vi "XPS Controller.vi"(4 "Axis 2":string="Group7", 5 "Axis 1":string="Group2", 7 "Controller Address":string="192.168.254.254", 9 "Axis 2 \ninverted?":bool=TRUE, 10 "Axis 1 \ninverted?":bool=TRUE) -> ()   [LabVIEW 2016]
uses:
  <vilib>/Utility/miscctls.llb/LVMinMaxIncTypeDef.ctl
panel:
  in  "Data Entry Limits":T1
  in  "Axis Initial Parameters":T2={"Velocity (units/seconds)"=1.0, "Acceleration (units/seconds²)"=20.0, "Minimum Jerk Time (seconds)"=0.005, "Maximum Jerk Time (seconds)"=0.009} {"Maximum Jerk Time (seconds)" format="%.6e"; "Minimum Jerk Time (seconds)" format="%.6e"; "Acceleration (units/seconds²)" format="%.6e"; "Velocity (units/seconds)" format="%.6e"}
  in  "Mode selector":bool
  in  "Axis 2 Velocity (slow)\nmm/s":dbl=1.0 min=0.0 max=10.0 step=0.0001
  in  "Axis 2 Velocity (fast)\nmm/s":dbl=5.0 min=0.0 max=10.0 step=0.0001
  in  "Velocity (slow)":dbl=1.0 min=0.0 max=5.0 step=0.0001
  in  "Velocity (fast)":dbl=5.0 min=0.0 max=5.0 step=0.0001
  in  "Refresh Time":u32=100 min=50 max=10000 step=1
  in  "Tab Control":enum32{"JOG MODE", "MOVE MODE"}(tab)
  in  "Axis 1 negative":bool
  in  "Axis 1 negative fast":bool
  in  "Axis 1 Positive":bool
  in  "Axis 1 Positive fast":bool
  in  "Axis 2 negative":bool
  in  "Axis 2 negative fast":bool
  in  "Axis 2 Positive":bool
  in  "Axis 2 Positive fast":bool
  in  "Absolute":dbl=5.0 min=0.0 max=50.0
  in  "Absolute Axis 2":dbl=5.0 min=-75.0 max=75.0
  in  "Axis 1 move absolute":bool
  in  "Axis 2 move absolute":bool
  in  "Relative":dbl=1.0 min=-50.0 max=50.0
  in  "Relative Axis 2":dbl=1.0 min=-150.0 max=150.0
  in  "Axis 1 move relative":bool
  in  "Axis 2 move relative":bool
  out "Axis 1 Model":string
  out "Axis 2 Model":string
  in  "stop 2":bool
  out "Axis 2 position":dbl format="%.10f"
  out "Axis 2 Status":string
  out "Axis 1 position":dbl format="%.10f"
  out "Axis 1 Status":string
  in  "Motion parameter":T3={"Velocity (units/s)"=5.0, "Acceleration (units/s²)"=20.0} {"Acceleration (units/s²)" format="%.6f"; "Velocity (units/s)" format="%.6f"}
  in  "stop":bool
  # "Axis 1"
  # "Axis 2"
  # "msec"
  # "Axis 1"
  # "Axis 2"
  # "Axis 1"
  # "Axis 2"
  # "Absolute"
  # "Relative"
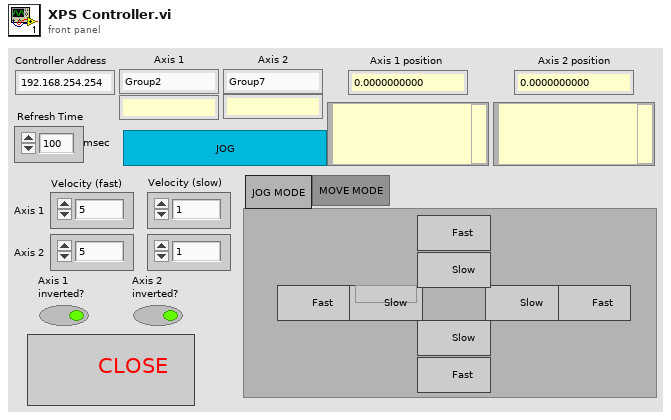
[diagram p1: front panel]
types:
  T1 = typedef "LVMinMaxIncTypeDef.ctl" = cluster{"Minimum":dbl, "Maximum":dbl, "Increment":dbl}
  T2 = cluster{"Velocity (units/seconds)":dbl, "Acceleration (units/seconds²)":dbl, "Minimum Jerk Time (seconds)":dbl, "Maximum Jerk Time (seconds)":dbl}
  T3 = cluster{"Velocity (units/s)":dbl, "Acceleration (units/s²)":dbl}
  T4 = enum32{"Page Enabled", "Page Disabled", "Page Disabled & Grayed"}
  T5 = cluster{"connection TCP":refnum<k5>, "LogTo File":bool, "Log File refnum":refnum<file>, "no error if error log":bool}
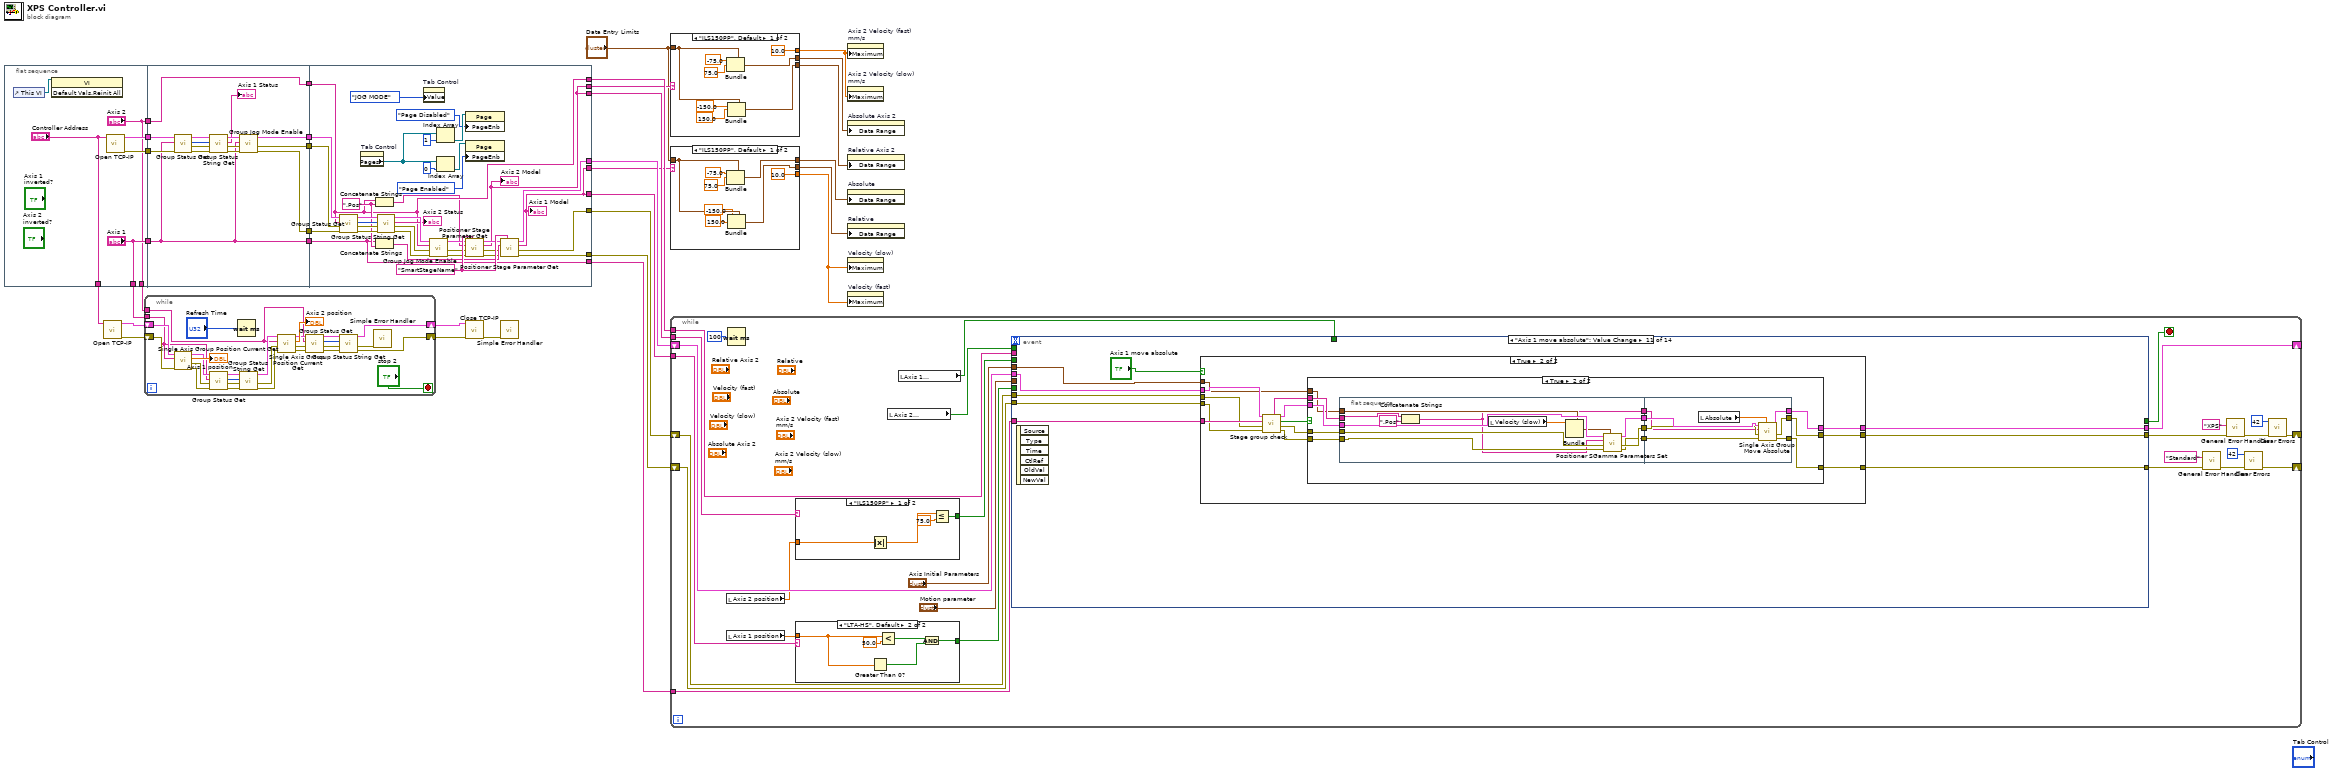
[diagram p0: block diagram]
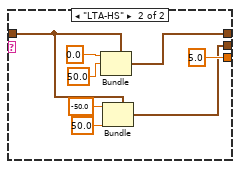
[diagram p2: hidden frame]
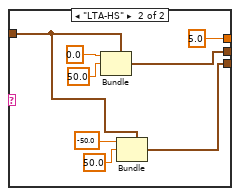
[diagram p3: hidden frame]
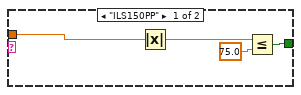
[diagram p4: hidden frame]
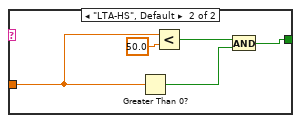
[diagram p5: hidden frame]
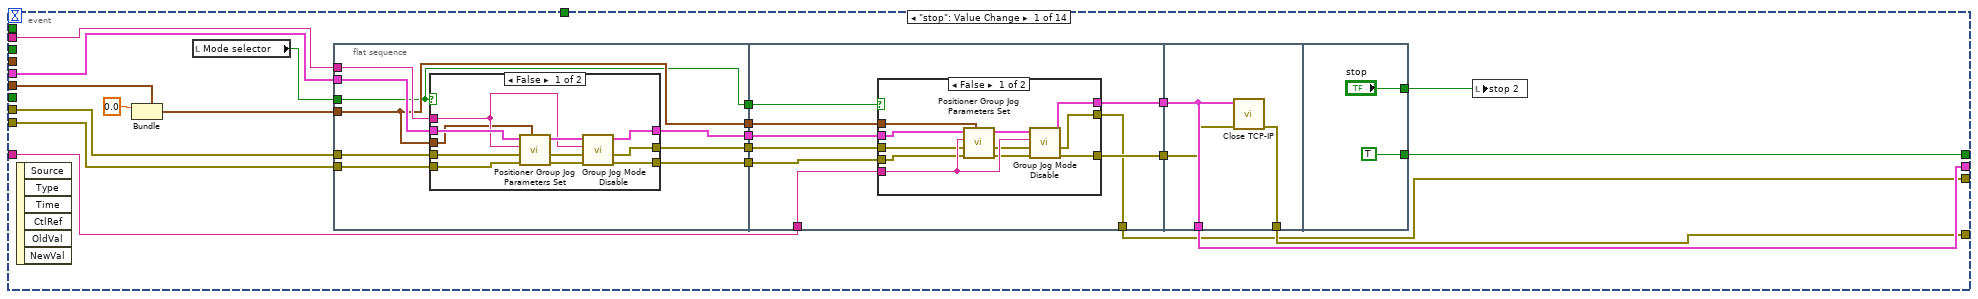
[diagram p6: hidden frame]
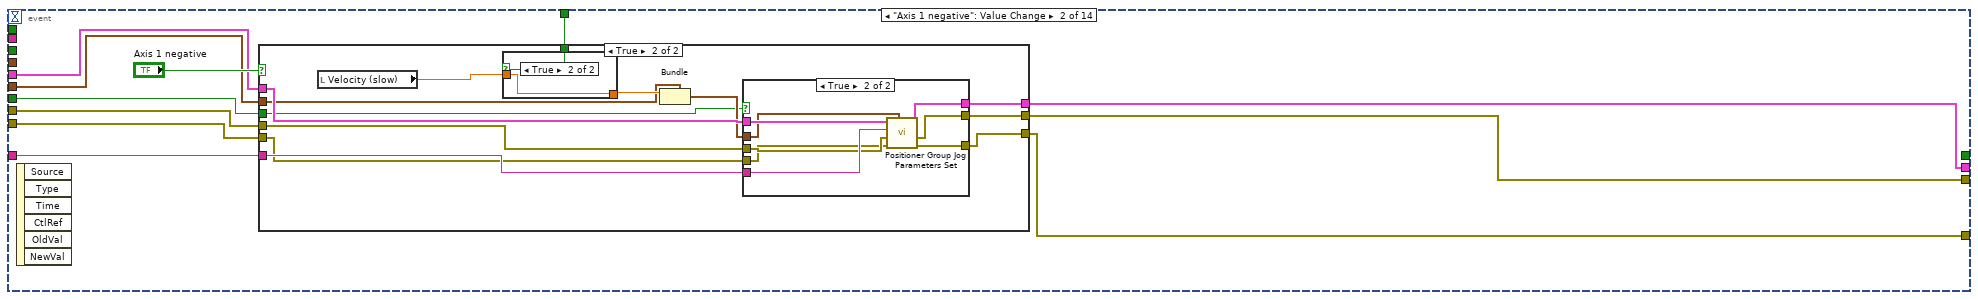
[diagram p9: hidden frame]
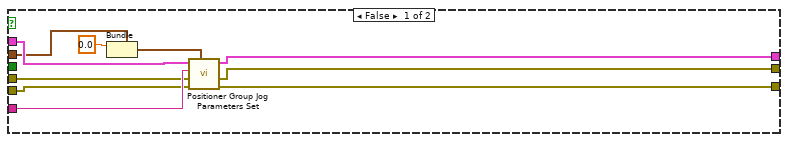
[diagram p10: hidden frame]
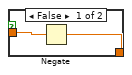
[diagram p11: hidden frame]
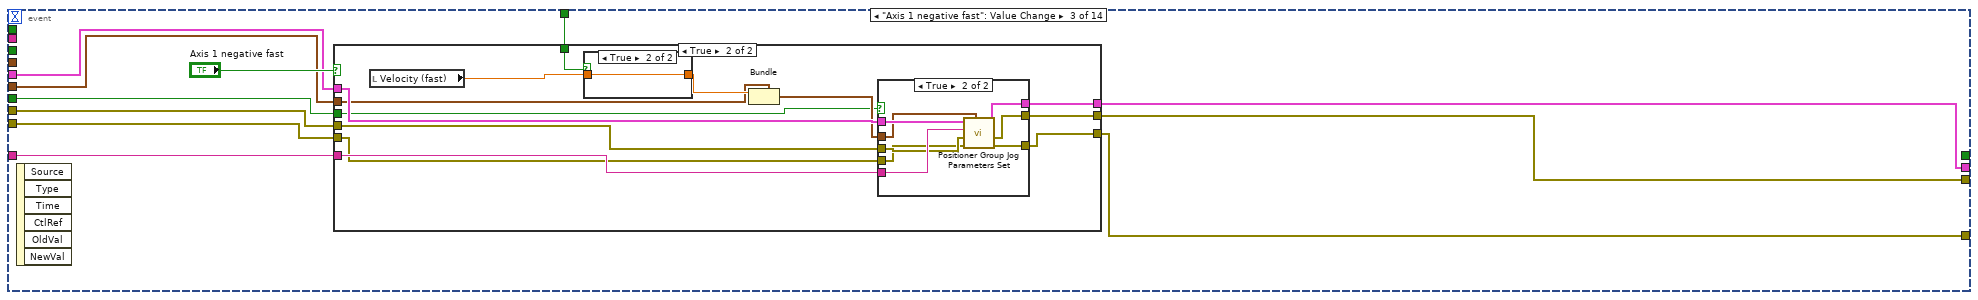
[diagram p13: hidden frame]
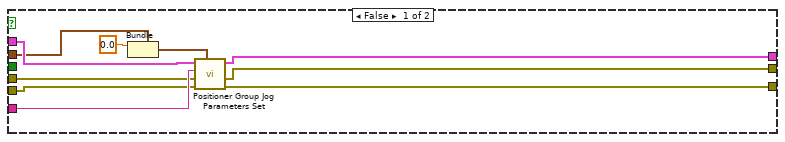
[diagram p14: hidden frame]
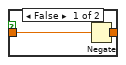
[diagram p15: hidden frame]
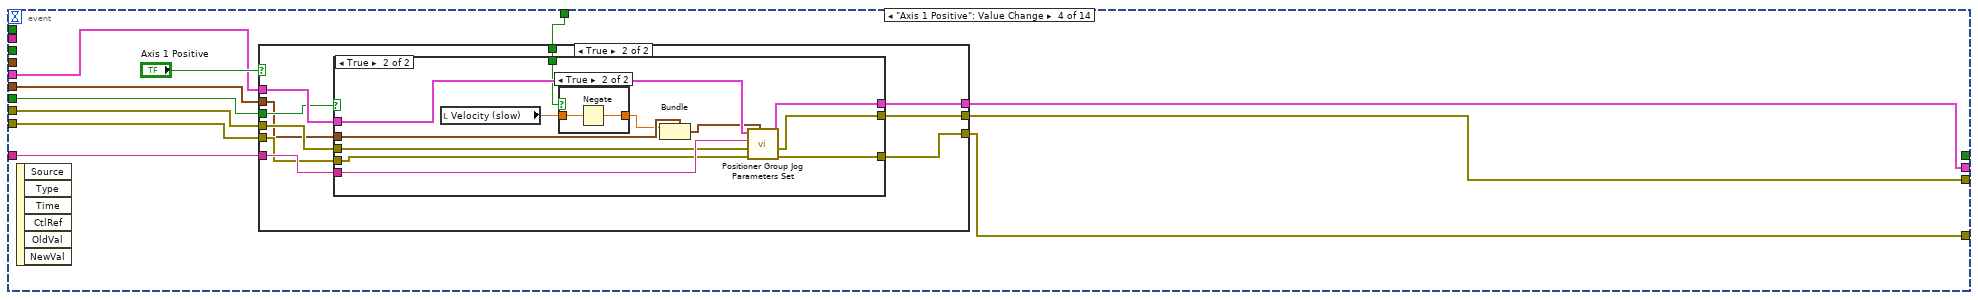
[diagram p17: hidden frame]
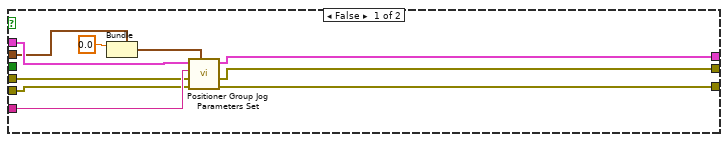
[diagram p18: hidden frame]
diagram:
  n1 = flat-sequence {
    tunnel: ["Axis 1"] -> w30
    tunnel: [w38] -> w29
    tunnel: [w37] -> w28
    tunnel: ["Axis 2"] -> w27
    tunnel: ["Controller Address"] -> w21
    tunnel: ["Axis 1"] -> w16
    tunnel: ["Axis 2"] -> w15
    tunnel: [w54] -> w33
    tunnel: [w53] -> w32
    tunnel: [w52] -> w31
    tunnel: w30 -> [w41]
    tunnel: w29 -> [w47]
    tunnel: w28 -> [w46]
    tunnel: w27 -> [w40]
    tunnel: [w40] -> w26
    tunnel: [w41] -> w24
    tunnel: w33 -> [w87]
    tunnel: w32 -> [w81]
    tunnel: w31 -> [w82]
    tunnel: w26 -> [w73]
    tunnel: w24 -> [w74]
    tunnel: [w65] -> w13
    tunnel: [w76] -> w25
    tunnel: [w74] -> w22
    tunnel: [w73] -> w23
    tunnel: [w68] -> w12
    tunnel: [w63] -> w11
    tunnel: [w64] -> w10
    tunnel: [w64] -> w9
    tunnel: [w63] -> w8
    frame #0 {
      n2 = control-ref of="This VI"() -> (w39:refnum<vi>)
      n3 = invoke class="VI" method="Default Vals.Reinit All"(reference=w39) -> ()  [unwired: 2 in, 3 out]
      n4 = call <userlib>:"Open TCP-IP.vi"("IP address"="Controller Address") -> ("error out"=w38:errorcluster, "Connection ID"=w37:T5)  [unwired: 5 in, 4 out]
    }
    frame #1 {
      n5 = call <userlib>:"Group Status Get.vi"("error in (no error)"=w47, "Group Name (250 c max)"=w41, "connection ID in"=w46) -> ("error out"=w50:errorcluster, "XPS error out"=w51:errorcluster, "Status"=w49:i32, "connection ID out"=w45:T5)  [unwired: 5 in]
      n6 = call <userlib>:"Group Status String Get.vi"("error in (no error)"=w50, "XPS error in (no error)"=w51, "Status #"=w49, "connection ID in"=w45) -> ("error out"=w44:errorcluster, "XPS error out"=w43:errorcluster, "Group Status String"=→"Axis 1 Status":string, "connection ID out"=w48:T5)  [unwired: 4 in]
      n7 = call <userlib>:"Group Jog Mode Enable.vi"("error in (no error)"=w44, "XPS error in (no error)"=w43, "Group Name (250 c max)"=w41, "connection ID in"=w48) -> ("error out"=w52:errorcluster, "XPS error out"=w53:errorcluster, "connection ID out"=w54:T5)  [unwired: 5 in]
    }
    frame #2 {
      w75 = ".Pos" ("string")
      w79 = "SmartStageName" ("Parameter Name (250 c max)")
      n8 = call <userlib>:"Group Status Get.vi"("error in (no error)"=w82, "XPS error in (no error)"=w81, "Group Name (250 c max)"=w73, "connection ID in"=w87) -> ("error out"=w89:errorcluster, "XPS error out"=w90:errorcluster, "Status"=w88:i32, "connection ID out"=w86:T5)  [unwired: 4 in]
      n9 = property on="Tab Control" class="TabCtl (strict)"() -> ("Pages"=w56:refnum<vi>[])  [unwired: 2 in, 2 out]
      n10 = Concatenate Strings(w73, w75) -> (w72:string)
      n11 = Concatenate Strings(w74, w75) -> (w71:string)
      n12 = call <userlib>:"Group Status String Get.vi"("error in (no error)"=w89, "XPS error in (no error)"=w90, "Status #"=w88, "connection ID in"=w86) -> ("error out"=w84:errorcluster, "XPS error out"=w83:errorcluster, "Group Status String"=→"Axis 2 Status":string, "connection ID out"=w85:T5)  [unwired: 4 in]
      n13 = property on="Tab Control" class="TabCtl (strict)"("Value"=enum32{"JOG MODE", "MOVE MODE"}."JOG MODE" ("Tab Control")) -> ()  [unwired: 2 in, 2 out]
      n14 = call <userlib>:"Group Jog Mode Enable.vi"("error in (no error)"=w84, "XPS error in (no error)"=w83, "Group Name (250 c max)"=w73, "connection ID in"=w85) -> ("error out"=w70:errorcluster, "XPS error out"=w67:errorcluster, "connection ID out"=w78:T5)  [unwired: 5 in]
      n15 = Index Array(array=w56, index=1) -> (element=w58:refnum<vi>)
      n16 = Index Array(array=w56, index=0) -> (element=w60:refnum<vi>)
      n17 = property class="Page"(reference=w58, "PageEnb"=T4."Page Disabled" ("Page Enabled State")) -> ()  [unwired: 1 in, 2 out]
      n18 = property class="Page"(reference=w60, "PageEnb"=T4."Page Enabled" ("Page Enabled State")) -> ()  [unwired: 1 in, 2 out]
      n19 = call <userlib>:"Positioner Stage Parameter Get.vi"("Parameter Name (250 c max)"=w79, "error in (no error)"=w70, "XPS error in (no error)"=w67, "Positioner Name (250 c max)"=w72, "connection ID in"=w78) -> ("error out"=w69:errorcluster, "XPS error out"=w66:errorcluster, "Parameter Value"=w64:string, "connection ID out"=w77:T5)  [unwired: 3 in]
      "Axis 2 Model" <- w64
      n20 = call <userlib>:"Positioner Stage Parameter Get.vi"("Parameter Name (250 c max)"=w79, "error in (no error)"=w69, "XPS error in (no error)"=w66, "Positioner Name (250 c max)"=w71, "connection ID in"=w77) -> ("error out"=w68:errorcluster, "XPS error out"=w65:errorcluster, "Parameter Value"=w63:string, "connection ID out"=w76:T5)  [unwired: 3 in]
      "Axis 1 Model" <- w63
    }
  }
  n21 = call <userlib>:"Open TCP-IP.vi"("IP address"=w21) -> ("error out"=w19:errorcluster, "Connection ID"=w20:T5)  [unwired: 5 in, 4 out]
  n22 = while {
    shift-right: [w93] -> w18
    shift-left: w20 -> [w118]
    shift-right: [w92] -> w17
    shift-left: w19 -> [w117]
    tunnel: w16 -> [w109]
    tunnel: w15 -> [w96]
    stop <- "stop 2" stop-if-true
    n23 = call <userlib>:"Single Axis Group Position Current Get.vi"("error in (no error)"=w117, "SingleAxis Group  Name (250 c max)"=w109, "connection ID in"=w118) -> ("error out"=w108:errorcluster, "XPS error out"=w107:errorcluster, "Current Position (units)"=→"Axis 1 position":dbl, "connection ID out"=w112:T5)  [unwired: 5 in]
    n24 = call <userlib>:"Group Status Get.vi"("error in (no error)"=w108, "XPS error in (no error)"=w107, "Group Name (250 c max)"=w109, "connection ID in"=w112) -> ("error out"=w105:errorcluster, "XPS error out"=w106:errorcluster, "Status"=w110:i32, "connection ID out"=w111:T5)  [unwired: 4 in]
    n25 = Wait (ms)(milliseconds to wait="Refresh Time") -> ()  [unwired: 1 out]
    n26 = call <userlib>:"Group Status String Get.vi"("error in (no error)"=w105, "XPS error in (no error)"=w106, "Status #"=w110, "connection ID in"=w111) -> ("error out"=w102:errorcluster, "XPS error out"=w103:errorcluster, "connection ID out"=w104:T5)  [unwired: 4 in, 1 out]
    n27 = call <userlib>:"Single Axis Group Position Current Get.vi"("error in (no error)"=w102, "XPS error in (no error)"=w103, "SingleAxis Group  Name (250 c max)"=w96, "connection ID in"=w104) -> ("error out"=w99:errorcluster, "XPS error out"=w100:errorcluster, "Current Position (units)"=→"Axis 2 position":dbl, "connection ID out"=w101:T5)  [unwired: 4 in]
    n28 = call <userlib>:"Group Status Get.vi"("error in (no error)"=w99, "XPS error in (no error)"=w100, "Group Name (250 c max)"=w96, "connection ID in"=w101) -> ("error out"=w97:errorcluster, "XPS error out"=w98:errorcluster, "Status"=w94:i32, "connection ID out"=w95:T5)  [unwired: 4 in]
    n29 = call <userlib>:"Group Status String Get.vi"("error in (no error)"=w97, "XPS error in (no error)"=w98, "Status #"=w94, "connection ID in"=w95) -> ("error out"=w92:errorcluster, "XPS error out"=w91:errorcluster, "connection ID out"=w93:T5)  [unwired: 4 in, 1 out]
    n30 = call <vilib>:"Simple Error Handler.vi"("error in (no error)"=w91) -> ()  [unwired: 4 in, 5 out]
  }
  n31 = call <userlib>:"Close TCP-IP.vi"("error in (no error)"=w17, "connection ID in"=w18) -> ("Error out"=w14:errorcluster)  [unwired: 9 in]
  n32 = call <vilib>:"Simple Error Handler.vi"("error in (no error)"=w14) -> ()  [unwired: 4 in, 5 out]
  n33 = case shown="\"ILS150PP\", Default" w9 {
    tunnel: [10.0 5.0] -> w7
    tunnel: "Data Entry Limits" -> [w122 w129]
    tunnel: [w123 w131] -> w4
    tunnel: [w120 w127] -> w3
    frame "ILS150PP", Default {
      n34 = Bundle(cluster=w122, "Minimum"=-75.0, "Maximum"=75.0) -> (w123:T1)  [unwired: 1 in]
      n35 = Bundle(cluster=w122, "Minimum"=-150.0, "Maximum"=150.0) -> (w120:T1)  [unwired: 1 in]
    }
    frame "LTA-HS" {
      n36 = Bundle(cluster=w129, "Minimum"=0.0, "Maximum"=50.0) -> (w131:T1)  [unwired: 1 in]
      n37 = Bundle(cluster=w129, "Minimum"=-50.0, "Maximum"=50.0) -> (w127:T1)  [unwired: 1 in]
    }
  }
  n38 = case shown="\"ILS150PP\", Default" w8 {
    tunnel: [10.0 5.0] -> w6
    tunnel: "Data Entry Limits" -> [w139 w146]
    tunnel: [w136 w143] -> w1
    tunnel: [w137 w147] -> w2
    frame "ILS150PP", Default {
      n39 = Bundle(cluster=w139, "Minimum"=-75.0, "Maximum"=75.0) -> (w137:T1)  [unwired: 1 in]
      n40 = Bundle(cluster=w139, "Minimum"=-150.0, "Maximum"=150.0) -> (w136:T1)  [unwired: 1 in]
    }
    frame "LTA-HS" {
      n41 = Bundle(cluster=w146, "Minimum"=0.0, "Maximum"=50.0) -> (w147:T1)  [unwired: 1 in]
      n42 = Bundle(cluster=w146, "Minimum"=-50.0, "Maximum"=50.0) -> (w143:T1)  [unwired: 1 in]
    }
  }
  n43 = while {
    shift-right: [w177] -> _
    shift-left: w25 -> [w178]
    tunnel: w23 -> [w176]
    tunnel: w22 -> [w175]
    shift-right: [w161] -> _
    shift-left: w12 -> [w168]
    shift-right: [w164] -> _
    shift-left: w13 -> [w169]
    tunnel: w11 -> [w156]
    tunnel: w10 -> [w155]
    stop <- w171 stop-if-true
    n44 = local read "Axis 2 position"() -> (w157:dbl)
    n45 = local read "Axis 1 position"() -> (w160:dbl)
    n46 = Wait (ms)(milliseconds to wait=u32 100) -> ()  [unwired: 1 out]
    n47 = case shown="\"ILS150PP\"" w155 {
      tunnel: w157 -> [w189 w194]
      tunnel: [w190 w192] -> w158
      frame "ILS150PP" {
        n48 = Absolute Value(x=w189) -> (abs(x)=w188:dbl)
        n49 = Less Or Equal?(x=w188, y=75.0) -> (x <= y?=w190:bool)
      }
      frame "LTA-HS", Default {
        n50 = Greater Than 0?(x=w194) -> (x > 0?=w193:bool)
        n51 = Less?(x=w194, y=50.0) -> (x < y?=w196:bool)
        n52 = And(x=w196, y=w193) -> (x .and. y?=w192:bool)
      }
    }
    n53 = case shown="\"LTA-HS\", Default" w156 {
      tunnel: w160 -> [w181 w185]
      tunnel: [w179 w183] -> w159
      frame "ILS150PP" {
        n54 = Absolute Value(x=w181) -> (abs(x)=w180:dbl)
        n55 = Less Or Equal?(x=w180, y=75.0) -> (x <= y?=w179:bool)
      }
      frame "LTA-HS", Default {
        n56 = Greater Than 0?(x=w185) -> (x > 0?=w184:bool)
        n57 = Less?(x=w185, y=50.0) -> (x < y?=w187:bool)
        n58 = And(x=w187, y=w184) -> (x .and. y?=w183:bool)
      }
    }
    n59 = local read "Axis 2 \ninverted?"() -> (w151:bool)
    n60 = local read "Axis 1 \ninverted?"() -> (w152:bool)
    n61 = event shown="[10] \"Axis 1 move absolute\": Value Change" {
      selector: _ -> [_ _ _ _ _ _ _ _ _ _ _ _ _ _]
      dyn-events: _ -> [_ _ _ _ _ _ _ _ _ _ _ _ _ _]
      timeout: _ -> [_ _ _ _ _ _ _ _ _ _ _ _ _ _]
      tunnel: [w202 w275 w323 w371 w423 w470 w517 w565 w614 w658 w823 w883 w954 w1022] -> w172
      tunnel: w178 -> [w217 w278 w326 w374 w424 w472 w520 w568 w617 w665 w829 w890 w961 w1030]
      tunnel: [w216 w277 w325 w373 w421 w469 w519 w567 w616 w660 w825 w885 w956 w1024] -> w177
      tunnel: [w201 w276 w324 w372 w422 w471 w518 w566 w615 w659 w824 w884 w955 w1023] -> w173
      tunnel: w176 -> [w211 _ _ _ _ w468 w516 w564 w613 w661 _ _ w959 w1027]
      tunnel: w175 -> [w210 w274 w322 w370 w419 _ _ _ _ w664 w828 w887 _ _]
      tunnel: [w209 _ _ _ _ _ _ _ _ _ _ _ _ _] -> w171
      tunnel: w169 -> [w207 w273 w321 w369 w418 w467 w515 w563 w612 w663 w827 w889 w960 w1029]
      tunnel: w168 -> [w203 w272 w320 w368 w417 w466 w514 w562 w611 w662 w826 w888 w958 w1028]
      tunnel: w158 -> [_ _ _ _ _ w465 w513 w561 w610 _ _ _ _ _]
      tunnel: w159 -> [_ w271 w319 w367 w416 _ _ _ _ _ _ _ _ _]
      tunnel: "Axis Initial Parameters" -> [_ _ _ _ _ _ _ _ _ _ w822 w891 w962 w1026]
      tunnel: "Motion parameter" -> [w200 w270 w318 w366 w415 w464 w512 w560 w609 w657 _ _ _ _]
      tunnel: w152 -> [_ w269 w317 w365 w414 _ _ _ _ _ _ w882 _ _]
      tunnel: w151 -> [_ _ _ _ _ w463 w511 w559 w608 _ _ _ w953 _]
      event "stop": Value Change {
        n62 = event-data() -> ()  [unwired: 1 in, 6 out]
        n63 = Bundle(cluster=w200, "Velocity (units/s)"=0.0) -> (w212:T3)  [unwired: 1 in]
        n64 = local read "Mode selector"() -> (w198:bool)
        n65 = flat-sequence {
          tunnel: w217 -> [w226]
          tunnel: [w225] -> w214
          tunnel: w212 -> [w219]
          tunnel: w211 -> [w224]
          tunnel: w207 -> [w223]
          tunnel: [w222] -> w206
          tunnel: [w221] -> w204
          tunnel: w203 -> [w220]
          tunnel: [w219] -> w199
          tunnel: w198 -> [w218]
          tunnel: [w218] -> w197
          tunnel: [w248] -> w215
          tunnel: w214 -> [w249]
          tunnel: w210 -> [w247]
          tunnel: w206 -> [w246]
          tunnel: [w245] -> w205
          tunnel: w204 -> [w244]
          tunnel: [w243] -> w201
          tunnel: w199 -> [w242]
          tunnel: w197 -> [w241]
          tunnel: [w266] -> w216
          tunnel: w215 -> [w266]
          tunnel: w205 -> [w265]
          tunnel: [w264] -> w202
          tunnel: [TRUE] -> w209
          tunnel: ["stop"] -> w208
          frame #0 {
            n66 = case shown="False" w218 {
              tunnel: w226 -> [w236 w240]
              tunnel: [w235 w240] -> w225
              tunnel: w224 -> [w234 _]
              tunnel: w223 -> [w233 w239]
              tunnel: [w231 w239] -> w222
              tunnel: [w230 w238] -> w221
              tunnel: w220 -> [w228 w238]
              tunnel: w219 -> [w227 _]
              frame False {
                n67 = call <userlib>:"Positioner Group Jog Parameters Set.vi"("Group Jog parameters"=w227, "error in (no error)"=w228, "XPS error in (no error)"=w233, "Positioner Name (250 c max)"=w234, "connection ID in"=w236) -> ("error out"=w229:errorcluster, "XPS error out"=w232:errorcluster, "connection ID out"=w237:T5)  [unwired: 4 in]
                n68 = call <userlib>:"Group Jog Mode Disable.vi"("error in (no error)"=w229, "XPS error in (no error)"=w232, "Group Name (250 c max)"=w234, "connection ID in"=w237) -> ("error out"=w230:errorcluster, "XPS error out"=w231:errorcluster, "connection ID out"=w235:T5)  [unwired: 5 in]
              }
              frame True {
              }
            }
          }
          frame #1 {
            n69 = case shown="False" w241 {
              tunnel: w249 -> [w260 w263]
              tunnel: [w258 w263] -> w248
              tunnel: w247 -> [w257 _]
              tunnel: w246 -> [w256 w262]
              tunnel: [w254 w261] -> w245
              tunnel: w244 -> [w252 w261]
              tunnel: [w251 w262] -> w243
              tunnel: w242 -> [w250 _]
              frame False {
                n70 = call <userlib>:"Positioner Group Jog Parameters Set.vi"("Group Jog parameters"=w250, "error in (no error)"=w252, "XPS error in (no error)"=w256, "Positioner Name (250 c max)"=w257, "connection ID in"=w260) -> ("error out"=w253:errorcluster, "XPS error out"=w255:errorcluster, "connection ID out"=w259:T5)  [unwired: 4 in]
                n71 = call <userlib>:"Group Jog Mode Disable.vi"("error in (no error)"=w253, "XPS error in (no error)"=w255, "Group Name (250 c max)"=w257, "connection ID in"=w259) -> ("error out"=w254:errorcluster, "XPS error out"=w251:errorcluster, "connection ID out"=w258:T5)  [unwired: 5 in]
              }
              frame True {
              }
            }
          }
          frame #2 {
            n72 = call <userlib>:"Close TCP-IP.vi"("error in (no error)"=w265, "connection ID in"=w266) -> ("Error out"=w264:errorcluster)  [unwired: 9 in]
          }
          frame #3 {
          }
        }
        n73 = local write "stop 2"(w208) -> ()
      }
      event "Axis 1 negative": Value Change {
        n74 = event-data() -> ()  [unwired: 1 in, 6 out]
        n75 = case shown="True" "Axis 1 negative" {
          tunnel: w278 -> [w289 w302]
          tunnel: [w288 w301] -> w277
          tunnel: [w287 w300] -> w276
          tunnel: [w286 w299] -> w275
          tunnel: w274 -> [w285 w298]
          tunnel: w273 -> [w283 w296]
          tunnel: w272 -> [w282 w295]
          tunnel: w271 -> [_ w294]
          tunnel: w270 -> [w281 w291]
          tunnel: w269 -> [_ w290]
          frame False {
            n76 = Bundle(cluster=w281, "Velocity (units/s)"=0.0) -> (w280:T3)  [unwired: 1 in]
            n77 = call <userlib>:"Positioner Group Jog Parameters Set.vi"("Group Jog parameters"=w280, "error in (no error)"=w282, "XPS error in (no error)"=w283, "Positioner Name (250 c max)"=w285, "connection ID in"=w289) -> ("error out"=w286:errorcluster, "XPS error out"=w287:errorcluster, "connection ID out"=w288:T5)  [unwired: 4 in]
          }
          frame True {
            n78 = local read "Velocity (slow)"() -> (w293:dbl)
            n79 = case shown="True" w290 {
              tunnel: w293 -> [w304 w305]
              tunnel: [w303 w305] -> w292
              frame False {
                n80 = Negate(x=w304) -> (-x=w303:dbl)
              }
              frame True {
              }
            }
            n81 = Bundle(cluster=w291, "Velocity (units/s)"=w292) -> (w297:T3)  [unwired: 1 in]
            n82 = case shown="True" w294 {
              tunnel: w302 -> [w308 w316]
              tunnel: [w308 w315] -> w301
              tunnel: [w307 w314] -> w300
              tunnel: [w306 w313] -> w299
              tunnel: w298 -> [_ w312]
              tunnel: w297 -> [_ w311]
              tunnel: w296 -> [w307 w310]
              tunnel: w295 -> [w306 w309]
              frame False {
              }
              frame True {
                n83 = call <userlib>:"Positioner Group Jog Parameters Set.vi"("Group Jog parameters"=w311, "error in (no error)"=w309, "XPS error in (no error)"=w310, "Positioner Name (250 c max)"=w312, "connection ID in"=w316) -> ("error out"=w313:errorcluster, "XPS error out"=w314:errorcluster, "connection ID out"=w315:T5)  [unwired: 4 in]
              }
            }
          }
        }
      }
      event "Axis 1 negative fast": Value Change {
        n84 = event-data() -> ()  [unwired: 1 in, 6 out]
        n85 = case shown="True" "Axis 1 negative fast" {
          tunnel: w326 -> [w337 w350]
          tunnel: [w336 w349] -> w325
          tunnel: [w335 w348] -> w324
          tunnel: [w334 w347] -> w323
          tunnel: w322 -> [w333 w346]
          tunnel: w321 -> [w331 w343]
          tunnel: w320 -> [w330 w342]
          tunnel: w319 -> [_ w341]
          tunnel: w318 -> [w329 w339]
          tunnel: w317 -> [_ w338]
          frame False {
            n86 = Bundle(cluster=w329, "Velocity (units/s)"=0.0) -> (w328:T3)  [unwired: 1 in]
            n87 = call <userlib>:"Positioner Group Jog Parameters Set.vi"("Group Jog parameters"=w328, "error in (no error)"=w330, "XPS error in (no error)"=w331, "Positioner Name (250 c max)"=w333, "connection ID in"=w337) -> ("error out"=w334:errorcluster, "XPS error out"=w335:errorcluster, "connection ID out"=w336:T5)  [unwired: 4 in]
          }
          frame True {
            n88 = local read "Velocity (fast)"() -> (w340:dbl)
            n89 = case shown="True" w338 {
              tunnel: [w352 w353] -> w345
              tunnel: w340 -> [w351 w353]
              frame False {
                n90 = Negate(x=w351) -> (-x=w352:dbl)
              }
              frame True {
              }
            }
            n91 = Bundle(cluster=w339, "Velocity (units/s)"=w345) -> (w344:T3)  [unwired: 1 in]
            n92 = case shown="True" w341 {
              tunnel: w350 -> [w354 w364]
              tunnel: [w354 w363] -> w349
              tunnel: [w355 w362] -> w348
              tunnel: [w356 w361] -> w347
              tunnel: w346 -> [_ w360]
              tunnel: w344 -> [_ w359]
              tunnel: w343 -> [w355 w358]
              tunnel: w342 -> [w356 w357]
              frame False {
              }
              frame True {
                n93 = call <userlib>:"Positioner Group Jog Parameters Set.vi"("Group Jog parameters"=w359, "error in (no error)"=w357, "XPS error in (no error)"=w358, "Positioner Name (250 c max)"=w360, "connection ID in"=w364) -> ("error out"=w361:errorcluster, "XPS error out"=w362:errorcluster, "connection ID out"=w363:T5)  [unwired: 4 in]
              }
            }
          }
        }
      }
      event "Axis 1 Positive": Value Change {
        n94 = event-data() -> ()  [unwired: 1 in, 6 out]
        n95 = case shown="True" "Axis 1 Positive" {
          tunnel: w374 -> [w385 w395]
          tunnel: [w384 w394] -> w373
          tunnel: [w383 w393] -> w372
          tunnel: [w382 w392] -> w371
          tunnel: w370 -> [w381 w391]
          tunnel: w369 -> [w379 w390]
          tunnel: w368 -> [w378 w389]
          tunnel: w367 -> [_ w388]
          tunnel: w366 -> [w377 w387]
          tunnel: w365 -> [_ w386]
          frame False {
            n96 = Bundle(cluster=w377, "Velocity (units/s)"=0.0) -> (w376:T3)  [unwired: 1 in]
            n97 = call <userlib>:"Positioner Group Jog Parameters Set.vi"("Group Jog parameters"=w376, "error in (no error)"=w378, "XPS error in (no error)"=w379, "Positioner Name (250 c max)"=w381, "connection ID in"=w385) -> ("error out"=w382:errorcluster, "XPS error out"=w383:errorcluster, "connection ID out"=w384:T5)  [unwired: 4 in]
          }
          frame True {
            n98 = case shown="True" w388 {
              tunnel: w395 -> [w396 w410]
              tunnel: [w396 w409] -> w394
              tunnel: [w398 w408] -> w393
              tunnel: [w397 w407] -> w392
              tunnel: w391 -> [_ w406]
              tunnel: w390 -> [w398 w405]
              tunnel: w389 -> [w397 w404]
              tunnel: w387 -> [_ w402]
              tunnel: w386 -> [_ w399]
              frame False {
              }
              frame True {
                n99 = local read "Velocity (slow)"() -> (w401:dbl)
                n100 = case shown="True" w399 {
                  tunnel: w401 -> [w411 w412]
                  tunnel: [w411 w413] -> w400
                  frame False {
                  }
                  frame True {
                    n101 = Negate(x=w412) -> (-x=w413:dbl)
                  }
                }
                n102 = Bundle(cluster=w402, "Velocity (units/s)"=w400) -> (w403:T3)  [unwired: 1 in]
                n103 = call <userlib>:"Positioner Group Jog Parameters Set.vi"("Group Jog parameters"=w403, "error in (no error)"=w404, "XPS error in (no error)"=w405, "Positioner Name (250 c max)"=w406, "connection ID in"=w410) -> ("error out"=w407:errorcluster, "XPS error out"=w408:errorcluster, "connection ID out"=w409:T5)  [unwired: 4 in]
              }
            }
          }
        }
      }
      event "Axis 1 Positive fast": Value Change {
        n104 = event-data() -> ()  [unwired: 1 in, 6 out]
        n105 = case shown="True" "Axis 1 Positive fast" {
          tunnel: w424 -> [w434 w444]
          tunnel: [w431 w441] -> w423
          tunnel: [w432 w442] -> w422
          tunnel: [w433 w443] -> w421
          tunnel: w419 -> [w430 w440]
          tunnel: w418 -> [w428 w438]
          tunnel: w417 -> [w427 w439]
          tunnel: w416 -> [_ w437]
          tunnel: w415 -> [w426 w436]
          tunnel: w414 -> [_ w435]
          frame False {
            n106 = Bundle(cluster=w426, "Velocity (units/s)"=0.0) -> (w425:T3)  [unwired: 1 in]
            n107 = call <userlib>:"Positioner Group Jog Parameters Set.vi"("Group Jog parameters"=w425, "error in (no error)"=w427, "XPS error in (no error)"=w428, "Positioner Name (250 c max)"=w430, "connection ID in"=w434) -> ("error out"=w431:errorcluster, "XPS error out"=w432:errorcluster, "connection ID out"=w433:T5)  [unwired: 4 in]
          }
          frame True {
            n108 = case shown="True" w437 {
              tunnel: w444 -> [w445 w459]
              tunnel: [w445 w458] -> w443
              tunnel: [w447 w457] -> w442
              tunnel: [w446 w456] -> w441
              tunnel: w440 -> [_ w455]
              tunnel: w439 -> [w446 w454]
              tunnel: w438 -> [w447 w453]
              tunnel: w436 -> [_ w451]
              tunnel: w435 -> [_ w448]
              frame False {
              }
              frame True {
                n109 = local read "Velocity (fast)"() -> (w450:dbl)
                n110 = case shown="True" w448 {
                  tunnel: w450 -> [w460 w461]
                  tunnel: [w460 w462] -> w449
                  frame False {
                  }
                  frame True {
                    n111 = Negate(x=w461) -> (-x=w462:dbl)
                  }
                }
                n112 = Bundle(cluster=w451, "Velocity (units/s)"=w449) -> (w452:T3)  [unwired: 1 in]
                n113 = call <userlib>:"Positioner Group Jog Parameters Set.vi"("Group Jog parameters"=w452, "error in (no error)"=w454, "XPS error in (no error)"=w453, "Positioner Name (250 c max)"=w455, "connection ID in"=w459) -> ("error out"=w456:errorcluster, "XPS error out"=w457:errorcluster, "connection ID out"=w458:T5)  [unwired: 4 in]
              }
            }
          }
        }
      }
      event "Axis 2 negative": Value Change {
        n114 = event-data() -> ()  [unwired: 1 in, 6 out]
        n115 = case shown="True" "Axis 2 negative" {
          tunnel: w472 -> [w483 w496]
          tunnel: [w481 w494] -> w471
          tunnel: [w480 w493] -> w470
          tunnel: [w482 w495] -> w469
          tunnel: w468 -> [w479 w492]
          tunnel: w467 -> [w477 w490]
          tunnel: w466 -> [w476 w489]
          tunnel: w465 -> [_ w488]
          tunnel: w464 -> [w475 w487]
          tunnel: w463 -> [_ w484]
          frame False {
            n116 = Bundle(cluster=w475, "Velocity (units/s)"=0.0) -> (w474:T3)  [unwired: 1 in]
            n117 = call <userlib>:"Positioner Group Jog Parameters Set.vi"("Group Jog parameters"=w474, "error in (no error)"=w476, "XPS error in (no error)"=w477, "Positioner Name (250 c max)"=w479, "connection ID in"=w483) -> ("error out"=w480:errorcluster, "XPS error out"=w481:errorcluster, "connection ID out"=w482:T5)  [unwired: 4 in]
          }
          frame True {
            n118 = local read "Axis 2 Velocity (slow)\nmm/s"() -> (w486:dbl)
            n119 = case shown="True" w484 {
              tunnel: [w498 w499] -> w485
              tunnel: w486 -> [w497 w499]
              frame False {
                n120 = Negate(x=w497) -> (-x=w498:dbl)
              }
              frame True {
              }
            }
            n121 = Bundle(cluster=w487, "Velocity (units/s)"=w485) -> (w491:T3)  [unwired: 1 in]
            n122 = case shown="True" w488 {
              tunnel: w496 -> [w502 w510]
              tunnel: [w502 w509] -> w495
              tunnel: [w501 w508] -> w494
              tunnel: [w500 w507] -> w493
              tunnel: w492 -> [_ w506]
              tunnel: w491 -> [_ w505]
              tunnel: w490 -> [w501 w504]
              tunnel: w489 -> [w500 w503]
              frame False {
              }
              frame True {
                n123 = call <userlib>:"Positioner Group Jog Parameters Set.vi"("Group Jog parameters"=w505, "error in (no error)"=w503, "XPS error in (no error)"=w504, "Positioner Name (250 c max)"=w506, "connection ID in"=w510) -> ("error out"=w507:errorcluster, "XPS error out"=w508:errorcluster, "connection ID out"=w509:T5)  [unwired: 4 in]
              }
            }
          }
        }
      }
      event "Axis 2 negative fast": Value Change {
        n124 = event-data() -> ()  [unwired: 1 in, 6 out]
        n125 = case shown="True" "Axis 2 negative fast" {
          tunnel: w520 -> [w531 w544]
          tunnel: [w530 w543] -> w519
          tunnel: [w529 w542] -> w518
          tunnel: [w528 w541] -> w517
          tunnel: w516 -> [w527 w540]
          tunnel: w515 -> [w525 w538]
          tunnel: w514 -> [w524 w537]
          tunnel: w513 -> [_ w536]
          tunnel: w512 -> [w523 w535]
          tunnel: w511 -> [_ w532]
          frame False {
            n126 = Bundle(cluster=w523, "Velocity (units/s)"=0.0) -> (w522:T3)  [unwired: 1 in]
            n127 = call <userlib>:"Positioner Group Jog Parameters Set.vi"("Group Jog parameters"=w522, "error in (no error)"=w524, "XPS error in (no error)"=w525, "Positioner Name (250 c max)"=w527, "connection ID in"=w531) -> ("error out"=w528:errorcluster, "XPS error out"=w529:errorcluster, "connection ID out"=w530:T5)  [unwired: 4 in]
          }
          frame True {
            n128 = local read "Axis 2 Velocity (fast)\nmm/s"() -> (w534:dbl)
            n129 = case shown="True" w532 {
              tunnel: [w546 w547] -> w533
              tunnel: w534 -> [w545 w547]
              frame False {
                n130 = Negate(x=w545) -> (-x=w546:dbl)
              }
              frame True {
              }
            }
            n131 = Bundle(cluster=w535, "Velocity (units/s)"=w533) -> (w539:T3)  [unwired: 1 in]
            n132 = case shown="True" w536 {
              tunnel: w544 -> [w550 w558]
              tunnel: [w550 w557] -> w543
              tunnel: [w549 w556] -> w542
              tunnel: [w548 w555] -> w541
              tunnel: w540 -> [_ w554]
              tunnel: w539 -> [_ w553]
              tunnel: w538 -> [w549 w552]
              tunnel: w537 -> [w548 w551]
              frame False {
              }
              frame True {
                n133 = call <userlib>:"Positioner Group Jog Parameters Set.vi"("Group Jog parameters"=w553, "error in (no error)"=w551, "XPS error in (no error)"=w552, "Positioner Name (250 c max)"=w554, "connection ID in"=w558) -> ("error out"=w555:errorcluster, "XPS error out"=w556:errorcluster, "connection ID out"=w557:T5)  [unwired: 4 in]
              }
            }
          }
        }
      }
      event "Axis 2 Positive": Value Change {
        n134 = event-data() -> ()  [unwired: 1 in, 6 out]
        n135 = case shown="True" "Axis 2 Positive" {
          tunnel: w568 -> [w579 w589]
          tunnel: [w578 w588] -> w567
          tunnel: [w577 w587] -> w566
          tunnel: [w576 w586] -> w565
          tunnel: w564 -> [w575 w585]
          tunnel: w563 -> [w572 w584]
          tunnel: w562 -> [w573 w583]
          tunnel: w561 -> [_ w582]
          tunnel: w560 -> [w571 w581]
          tunnel: w559 -> [_ w580]
          frame False {
            n136 = Bundle(cluster=w571, "Velocity (units/s)"=0.0) -> (w570:T3)  [unwired: 1 in]
            n137 = call <userlib>:"Positioner Group Jog Parameters Set.vi"("Group Jog parameters"=w570, "error in (no error)"=w573, "XPS error in (no error)"=w572, "Positioner Name (250 c max)"=w575, "connection ID in"=w579) -> ("error out"=w576:errorcluster, "XPS error out"=w577:errorcluster, "connection ID out"=w578:T5)  [unwired: 4 in]
          }
          frame True {
            n138 = case shown="True" w582 {
              tunnel: w589 -> [w592 w604]
              tunnel: [w592 w603] -> w588
              tunnel: [w591 w602] -> w587
              tunnel: [w590 w601] -> w586
              tunnel: w585 -> [_ w600]
              tunnel: w584 -> [w591 w599]
              tunnel: w583 -> [w590 w598]
              tunnel: w581 -> [_ w596]
              tunnel: w580 -> [_ w593]
              frame False {
              }
              frame True {
                n139 = local read "Axis 2 Velocity (slow)\nmm/s"() -> (w595:dbl)
                n140 = case shown="True" w593 {
                  tunnel: w595 -> [w605 w606]
                  tunnel: [w605 w607] -> w594
                  frame False {
                  }
                  frame True {
                    n141 = Negate(x=w606) -> (-x=w607:dbl)
                  }
                }
                n142 = Bundle(cluster=w596, "Velocity (units/s)"=w594) -> (w597:T3)  [unwired: 1 in]
                n143 = call <userlib>:"Positioner Group Jog Parameters Set.vi"("Group Jog parameters"=w597, "error in (no error)"=w598, "XPS error in (no error)"=w599, "Positioner Name (250 c max)"=w600, "connection ID in"=w604) -> ("error out"=w601:errorcluster, "XPS error out"=w602:errorcluster, "connection ID out"=w603:T5)  [unwired: 4 in]
              }
            }
          }
        }
      }
      event "Axis 2 Positive fast": Value Change {
        n144 = event-data() -> ()  [unwired: 1 in, 6 out]
        n145 = case shown="True" "Axis 2 Positive fast" {
          tunnel: w617 -> [w628 w638]
          tunnel: [w627 w635] -> w616
          tunnel: [w626 w636] -> w615
          tunnel: [w625 w637] -> w614
          tunnel: w613 -> [w624 w634]
          tunnel: w612 -> [w621 w633]
          tunnel: w611 -> [w622 w632]
          tunnel: w610 -> [_ w631]
          tunnel: w609 -> [w620 w630]
          tunnel: w608 -> [_ w629]
          frame False {
            n146 = Bundle(cluster=w620, "Velocity (units/s)"=0.0) -> (w619:T3)  [unwired: 1 in]
            n147 = call <userlib>:"Positioner Group Jog Parameters Set.vi"("Group Jog parameters"=w619, "error in (no error)"=w622, "XPS error in (no error)"=w621, "Positioner Name (250 c max)"=w624, "connection ID in"=w628) -> ("error out"=w625:errorcluster, "XPS error out"=w626:errorcluster, "connection ID out"=w627:T5)  [unwired: 4 in]
          }
          frame True {
            n148 = case shown="True" w631 {
              tunnel: w638 -> [w641 w653]
              tunnel: [w639 w652] -> w637
              tunnel: [w640 w651] -> w636
              tunnel: [w641 w650] -> w635
              tunnel: w634 -> [_ w649]
              tunnel: w633 -> [w640 w648]
              tunnel: w632 -> [w639 w647]
              tunnel: w630 -> [_ w645]
              tunnel: w629 -> [_ w642]
              frame False {
              }
              frame True {
                n149 = local read "Axis 2 Velocity (fast)\nmm/s"() -> (w644:dbl)
                n150 = case shown="True" w642 {
                  tunnel: w644 -> [w654 w655]
                  tunnel: [w654 w656] -> w643
                  frame False {
                  }
                  frame True {
                    n151 = Negate(x=w655) -> (-x=w656:dbl)
                  }
                }
                n152 = Bundle(cluster=w645, "Velocity (units/s)"=w643) -> (w646:T3)  [unwired: 1 in]
                n153 = call <userlib>:"Positioner Group Jog Parameters Set.vi"("Group Jog parameters"=w646, "error in (no error)"=w647, "XPS error in (no error)"=w648, "Positioner Name (250 c max)"=w649, "connection ID in"=w653) -> ("error out"=w652:errorcluster, "XPS error out"=w651:errorcluster, "connection ID out"=w650:T5)  [unwired: 4 in]
              }
            }
          }
        }
      }
      event "Mode selector": Value Change {
        n154 = event-data() -> ()  [unwired: 1 in, 6 out]
        n155 = case shown="False" "Mode selector" {
          tunnel: w665 -> [w681 w751]
          tunnel: w664 -> [w677 w749]
          tunnel: w663 -> [w680 w747]
          tunnel: w662 -> [w679 w746]
          tunnel: w661 -> [w678 w748]
          tunnel: [w684 w762] -> w660
          tunnel: [w683 w761] -> w659
          tunnel: [w682 w760] -> w658
          tunnel: w657 -> [_ w745]
          frame False {
            n156 = call "Stage group check.vi"("error in (no error)"=w679, "XPS error in (no error)"=w680, "Group Name (250 c max)"=w677, "connection ID in"=w681) -> ("error out"=w669:errorcluster, "XPS error out"=w670:errorcluster, "Stages ready?"=w667:bool, "connection ID out"=w674:T5, "Group Name (250 c max) 2"=w676:string)  [unwired: 3 in]
            n157 = call "Stage group check.vi"("error in (no error)"=w669, "XPS error in (no error)"=w670, "Group Name (250 c max)"=w678, "connection ID in"=w674) -> ("error out"=w671:errorcluster, "XPS error out"=w672:errorcluster, "Stages ready?"=w668:bool, "connection ID out"=w673:T5, "Group Name (250 c max) 2"=w675:string)  [unwired: 3 in]
            n158 = And(x=w667, y=w668) -> (x .and. y?=w685:bool)
            n159 = case shown="True" w685 {
              tunnel: [w686 w701] -> w684
              tunnel: [w687 w700] -> w683
              tunnel: [w688 w699] -> w682
              tunnel: w675 -> [_ w697]
              tunnel: w676 -> [_ w696]
              tunnel: w673 -> [w686 w695]
              tunnel: w672 -> [w687 w694]
              tunnel: w671 -> [w688 w693]
              frame False {
                n160 = One Button Dialog(message="Axes are not ready") -> ()  [unwired: 1 in, 1 out]
              }
              frame True {
                n161 = flat-sequence {
                  tunnel: [w710] -> w703
                  tunnel: [w709] -> w702
                  tunnel: [w708] -> w698
                  tunnel: w696 -> [w707]
                  tunnel: w695 -> [w706]
                  tunnel: w694 -> [w705]
                  tunnel: w693 -> [w704]
                  tunnel: w703 -> [w725]
                  tunnel: w702 -> [w724]
                  tunnel: w698 -> [w720]
                  tunnel: w697 -> [w719]
                  tunnel: [w723] -> w692
                  tunnel: [w722] -> w691
                  tunnel: [w721] -> w690
                  tunnel: [w742] -> w699
                  tunnel: [w743] -> w700
                  tunnel: [w744] -> w701
                  tunnel: w692 -> [w744]
                  tunnel: w691 -> [w743]
                  tunnel: w690 -> [w742]
                  frame #0 {
                    n162 = call <userlib>:"Group Status Get.vi"("error in (no error)"=w704, "XPS error in (no error)"=w705, "Group Name (250 c max)"=w707, "connection ID in"=w706) -> ("error out"=w717:errorcluster, "XPS error out"=w718:errorcluster, "Status"=w716:i32, "connection ID out"=w714:T5)  [unwired: 4 in]
                    n163 = call <userlib>:"Group Status String Get.vi"("error in (no error)"=w717, "XPS error in (no error)"=w718, "Status #"=w716, "connection ID in"=w714) -> ("error out"=w713:errorcluster, "XPS error out"=w712:errorcluster, "Group Status String"=w711:string, "connection ID out"=w715:T5)  [unwired: 4 in]
                    n164 = local write "Axis 1 Status"(w711) -> ()
                    n165 = call <userlib>:"Group Jog Mode Enable.vi"("error in (no error)"=w713, "XPS error in (no error)"=w712, "Group Name (250 c max)"=w707, "connection ID in"=w715) -> ("error out"=w710:errorcluster, "XPS error out"=w709:errorcluster, "connection ID out"=w708:T5)  [unwired: 5 in]
                  }
                  frame #1 {
                    n166 = call <userlib>:"Group Status Get.vi"("error in (no error)"=w725, "XPS error in (no error)"=w724, "Group Name (250 c max)"=w719, "connection ID in"=w720) -> ("error out"=w732:errorcluster, "XPS error out"=w733:errorcluster, "Status"=w731:i32, "connection ID out"=w729:T5)  [unwired: 4 in]
                    n167 = call <userlib>:"Group Status String Get.vi"("error in (no error)"=w732, "XPS error in (no error)"=w733, "Status #"=w731, "connection ID in"=w729) -> ("error out"=w728:errorcluster, "XPS error out"=w727:errorcluster, "Group Status String"=w726:string, "connection ID out"=w730:T5)  [unwired: 4 in]
                    n168 = local write "Axis 2 Status"(w726) -> ()
                    n169 = call <userlib>:"Group Jog Mode Enable.vi"("error in (no error)"=w728, "XPS error in (no error)"=w727, "Group Name (250 c max)"=w719, "connection ID in"=w730) -> ("error out"=w721:errorcluster, "XPS error out"=w722:errorcluster, "connection ID out"=w723:T5)  [unwired: 5 in]
                  }
                  frame #2 {
                    n170 = property on="Tab Control" class="TabCtl (strict)"() -> ("Pages"=w735:refnum<vi>[])  [unwired: 2 in, 2 out]
                    n171 = property on="Tab Control" class="TabCtl (strict)"("Value"=enum32{"JOG MODE", "MOVE MODE"}."JOG MODE" ("Tab Control")) -> ()  [unwired: 2 in, 2 out]
                    n172 = Index Array(array=w735, index=1) -> (element=w737:refnum<vi>)
                    n173 = Index Array(array=w735, index=0) -> (element=w739:refnum<vi>)
                    n174 = property class="Page"(reference=w737, "PageEnb"=T4."Page Disabled" ("Page Enabled State")) -> ()  [unwired: 1 in, 2 out]
                    n175 = property class="Page"(reference=w739, "PageEnb"=T4."Page Enabled" ("Page Enabled State")) -> ()  [unwired: 1 in, 2 out]
                  }
                }
              }
            }
          }
          frame True {
            w754 = 44
            n176 = call <userlib>:"Group Status Get.vi"("error in (no error)"=w746, "XPS error in (no error)"=w747, "Group Name (250 c max)"=w748, "connection ID in"=w751) -> ("error out"=w758:errorcluster, "XPS error out"=w757:errorcluster, "Status"=w755:i32, "connection ID out"=w759:T5)  [unwired: 4 in]
            n177 = call <userlib>:"Group Status Get.vi"("error in (no error)"=w758, "XPS error in (no error)"=w757, "Group Name (250 c max)"=w749, "connection ID in"=w759) -> ("error out"=w752:errorcluster, "XPS error out"=w753:errorcluster, "Status"=w756:i32, "connection ID out"=w750:T5)  [unwired: 4 in]
            n178 = Equal?(x=w755, y=w754) -> (x = y?=w764:bool)
            n179 = Equal?(x=w756, y=w754) -> (x = y?=w765:bool)
            n180 = And(x=w765, y=w764) -> (x .and. y?=w763:bool)
            n181 = case shown="False" w763 {
              tunnel: w750 -> [w781 w817]
              tunnel: w749 -> [w780 _]
              tunnel: w753 -> [w779 w819]
              tunnel: w752 -> [w778 w818]
              tunnel: w748 -> [w774 _]
              tunnel: [w773 w817] -> w762
              tunnel: [w772 w819] -> w761
              tunnel: [w771 w818] -> w760
              tunnel: w745 -> [w767 _]
              frame False {
                n182 = flat-sequence {
                  tunnel: w781 -> [w790]
                  tunnel: w780 -> [w787]
                  tunnel: w779 -> [w789]
                  tunnel: w778 -> [w788]
                  tunnel: [w786] -> w777
                  tunnel: [w785] -> w776
                  tunnel: [w784] -> w775
                  tunnel: w767 -> [w783]
                  tunnel: [w782] -> w766
                  tunnel: w777 -> [w802]
                  tunnel: w776 -> [w801]
                  tunnel: w775 -> [w800]
                  tunnel: w774 -> [w799]
                  tunnel: [w798] -> w770
                  tunnel: [w797] -> w769
                  tunnel: [w796] -> w768
                  tunnel: w766 -> [w795]
                  tunnel: [w814] -> w771
                  tunnel: [w815] -> w772
                  tunnel: [w816] -> w773
                  tunnel: w770 -> [w816]
                  tunnel: w769 -> [w815]
                  tunnel: w768 -> [w814]
                  frame #0 {
                    n183 = Bundle(cluster=w783, "Velocity (units/s)"=0.0) -> (w782:T3)  [unwired: 1 in]
                    n184 = call <userlib>:"Positioner Group Jog Parameters Set.vi"("Group Jog parameters"=w782, "error in (no error)"=w788, "XPS error in (no error)"=w789, "Positioner Name (250 c max)"=w787, "connection ID in"=w790) -> ("error out"=w791:errorcluster, "XPS error out"=w792:errorcluster, "connection ID out"=w793:T5)  [unwired: 4 in]
                    n185 = call <userlib>:"Group Jog Mode Disable.vi"("error in (no error)"=w791, "XPS error in (no error)"=w792, "Group Name (250 c max)"=w787, "connection ID in"=w793) -> ("error out"=w784:errorcluster, "XPS error out"=w785:errorcluster, "connection ID out"=w786:T5)  [unwired: 5 in]
                  }
                  frame #1 {
                    n186 = call <userlib>:"Positioner Group Jog Parameters Set.vi"("Group Jog parameters"=w795, "error in (no error)"=w800, "XPS error in (no error)"=w801, "Positioner Name (250 c max)"=w799, "connection ID in"=w802) -> ("error out"=w805:errorcluster, "XPS error out"=w804:errorcluster, "connection ID out"=w803:T5)  [unwired: 4 in]
                    n187 = call <userlib>:"Group Jog Mode Disable.vi"("error in (no error)"=w805, "XPS error in (no error)"=w804, "Group Name (250 c max)"=w799, "connection ID in"=w803) -> ("error out"=w796:errorcluster, "XPS error out"=w797:errorcluster, "connection ID out"=w798:T5)  [unwired: 5 in]
                  }
                  frame #2 {
                    n188 = property on="Tab Control" class="TabCtl (strict)"() -> ("Pages"=w807:refnum<vi>[])  [unwired: 2 in, 2 out]
                    n189 = Index Array(array=w807, index=1) -> (element=w809:refnum<vi>)
                    n190 = Index Array(array=w807, index=0) -> (element=w811:refnum<vi>)
                    n191 = property on="Tab Control" class="TabCtl (strict)"("Value"=enum32{"JOG MODE", "MOVE MODE"}."MOVE MODE" ("Tab Control")) -> ()  [unwired: 2 in, 2 out]
                    n192 = property class="Page"(reference=w809, "PageEnb"=T4."Page Enabled" ("Page Enabled State")) -> ()  [unwired: 1 in, 2 out]
                    n193 = property class="Page"(reference=w811, "PageEnb"=T4."Page Disabled" ("Page Enabled State")) -> ()  [unwired: 1 in, 2 out]
                  }
                }
              }
              frame True {
                n194 = One Button Dialog(message="Axes are still moving") -> ()  [unwired: 1 in, 1 out]
              }
            }
          }
        }
      }
      event "Axis 1 move absolute": Value Change {
        n195 = event-data() -> ()  [unwired: 1 in, 6 out]
        n196 = case shown="True" "Axis 1 move absolute" {
          tunnel: w829 -> [w832 w844]
          tunnel: w828 -> [_ w843]
          tunnel: w827 -> [w831 w842]
          tunnel: w826 -> [w830 w841]
          tunnel: [w832 w839] -> w825
          tunnel: [w831 w837] -> w824
          tunnel: [w830 w835] -> w823
          tunnel: w822 -> [_ w833]
          frame False {
          }
          frame True {
            n197 = call "Stage group check.vi"("error in (no error)"=w841, "XPS error in (no error)"=w842, "Group Name (250 c max)"=w843, "connection ID in"=w844) -> ("error out"=w836:errorcluster, "XPS error out"=w838:errorcluster, "Stages ready?"=w845:bool, "connection ID out"=w840:T5, "Group Name (250 c max) 2"=w834:string)  [unwired: 3 in]
            n198 = case shown="True" w845 {
              tunnel: w840 -> [w848 w861]
              tunnel: [w848 w852] -> w839
              tunnel: w838 -> [w847 w859]
              tunnel: [w847 w851] -> w837
              tunnel: w836 -> [w846 w858]
              tunnel: [w846 w850] -> w835
              tunnel: w834 -> [_ w860]
              tunnel: w833 -> [_ w857]
              frame False {
                n199 = One Button Dialog(message="Stage 1 is not ready") -> ()  [unwired: 1 in, 1 out]
              }
              frame True {
                n200 = flat-sequence {
                  tunnel: w861 -> [w873]
                  tunnel: w860 -> [w862]
                  tunnel: w859 -> [w872]
                  tunnel: w858 -> [w871]
                  tunnel: w857 -> [w870]
                  tunnel: [w867] -> w856
                  tunnel: [w866] -> w855
                  tunnel: [w865] -> w854
                  tunnel: [w863] -> w853
                  tunnel: w856 -> [w881]
                  tunnel: w855 -> [w880]
                  tunnel: w854 -> [w879]
                  tunnel: w853 -> [w878]
                  tunnel: [w877] -> w852
                  tunnel: [w876] -> w851
                  tunnel: [w875] -> w850
                  frame #0 {
                    n201 = Concatenate Strings(w862, ".Pos" ("string")) -> (w863:string)
                    n202 = local read "Velocity (slow)"() -> (w869:dbl)
                    n203 = Bundle(cluster=w870, "Velocity (units/seconds)"=w869) -> (w868:T2)  [unwired: 3 in]
                    n204 = call <userlib>:"Positioner SGamma Parameters Set.vi"("SGamma Parameters"=w868, "error in (no error)"=w871, "XPS error in (no error)"=w872, "Positioner Name (250 c max)"=w863, "connection ID in"=w873) -> ("error out"=w865:errorcluster, "XPS error out"=w866:errorcluster, "connection ID out"=w867:T5)  [unwired: 4 in]
                  }
                  frame #1 {
                    n205 = local read "Absolute"() -> (w874:dbl)
                    n206 = call <userlib>:"Single Axis Group Move Absolute.vi"("Target Position (units)"=w874, "error in (no error)"=w879, "XPS error in (no error)"=w880, "SingleAxis Group  Name (250 c max)"=w878, "connection ID in"=w881) -> ("error out"=w875:errorcluster, "XPS error out"=w876:errorcluster, "connection ID out"=w877:T5)  [unwired: 4 in]
                  }
                }
              }
            }
          }
        }
      }
      event "Axis 1 move relative": Value Change {
        n207 = event-data() -> ()  [unwired: 1 in, 6 out]
        n208 = case shown="True" "Axis 1 move relative" {
          tunnel: w890 -> [w894 w907]
          tunnel: w887 -> [_ w906]
          tunnel: w889 -> [w893 w905]
          tunnel: w888 -> [w892 w904]
          tunnel: [w894 w902] -> w885
          tunnel: [w893 w900] -> w884
          tunnel: [w892 w898] -> w883
          tunnel: w891 -> [_ w896]
          tunnel: w882 -> [_ w895]
          frame False {
          }
          frame True {
            n209 = call "Stage group check.vi"("error in (no error)"=w904, "XPS error in (no error)"=w905, "Group Name (250 c max)"=w906, "connection ID in"=w907) -> ("error out"=w899:errorcluster, "XPS error out"=w901:errorcluster, "Stages ready?"=w908:bool, "connection ID out"=w903:T5, "Group Name (250 c max) 2"=w897:string)  [unwired: 3 in]
            n210 = case shown="True" w908 {
              tunnel: w903 -> [w911 w926]
              tunnel: [w911 w917] -> w902
              tunnel: w901 -> [w910 w924]
              tunnel: [w910 w916] -> w900
              tunnel: w899 -> [w909 w923]
              tunnel: [w909 w915] -> w898
              tunnel: w897 -> [_ w925]
              tunnel: w896 -> [_ w922]
              tunnel: w895 -> [_ w914]
              frame False {
                n211 = One Button Dialog(message="Stage 1 is not ready") -> ()  [unwired: 1 in, 1 out]
              }
              frame True {
                n212 = flat-sequence {
                  tunnel: w926 -> [w939]
                  tunnel: w925 -> [w930]
                  tunnel: w924 -> [w938]
                  tunnel: w923 -> [w937]
                  tunnel: w922 -> [w936]
                  tunnel: [w934] -> w921
                  tunnel: [w933] -> w920
                  tunnel: [w932] -> w919
                  tunnel: [w929] -> w918
                  tunnel: w914 -> [w927]
                  tunnel: [w927] -> w913
                  tunnel: w921 -> [w949]
                  tunnel: w920 -> [w948]
                  tunnel: w919 -> [w947]
                  tunnel: w918 -> [w946]
                  tunnel: [w945] -> w917
                  tunnel: [w944] -> w916
                  tunnel: [w943] -> w915
                  tunnel: w913 -> [w940]
                  frame #0 {
                    n213 = local read "Velocity (slow)"() -> (w928:dbl)
                    n214 = Concatenate Strings(w930, ".Pos" ("string")) -> (w929:string)
                    n215 = Bundle(cluster=w936, "Velocity (units/seconds)"=w928) -> (w935:T2)  [unwired: 3 in]
                    n216 = call <userlib>:"Positioner SGamma Parameters Set.vi"("SGamma Parameters"=w935, "error in (no error)"=w937, "XPS error in (no error)"=w938, "Positioner Name (250 c max)"=w929, "connection ID in"=w939) -> ("error out"=w932:errorcluster, "XPS error out"=w933:errorcluster, "connection ID out"=w934:T5)  [unwired: 4 in]
                  }
                  frame #1 {
                    n217 = local read "Relative"() -> (w942:dbl)
                    n218 = case shown="True" w940 {
                      tunnel: w942 -> [w950 w951]
                      tunnel: [w950 w952] -> w941
                      frame False {
                      }
                      frame True {
                        n219 = Negate(x=w951) -> (-x=w952:dbl)
                      }
                    }
                    n220 = call <userlib>:"Single Axis Group Move Relative.vi"("Target Displacement (units)"=w941, "error in (no error)"=w947, "XPS error in (no error)"=w948, "SingleAxis Group  Name (250 c max)"=w946, "connection ID in"=w949) -> ("error out"=w943:errorcluster, "XPS error out"=w944:errorcluster, "connection ID out"=w945:T5)  [unwired: 4 in]
                  }
                }
              }
            }
          }
        }
      }
      event "Axis 2 move relative": Value Change {
        n221 = event-data() -> ()  [unwired: 1 in, 6 out]
        n222 = case shown="True" "Axis 2 move relative" {
          tunnel: w961 -> [w965 w978]
          tunnel: w959 -> [_ w977]
          tunnel: w960 -> [w964 w976]
          tunnel: w958 -> [w963 w975]
          tunnel: [w965 w973] -> w956
          tunnel: [w964 w971] -> w955
          tunnel: [w963 w969] -> w954
          tunnel: w962 -> [_ w967]
          tunnel: w953 -> [_ w966]
          frame False {
          }
          frame True {
            n223 = call "Stage group check.vi"("error in (no error)"=w975, "XPS error in (no error)"=w976, "Group Name (250 c max)"=w977, "connection ID in"=w978) -> ("error out"=w970:errorcluster, "XPS error out"=w972:errorcluster, "Stages ready?"=w979:bool, "connection ID out"=w974:T5, "Group Name (250 c max) 2"=w968:string)  [unwired: 3 in]
            n224 = case shown="True" w979 {
              tunnel: w974 -> [w982 w996]
              tunnel: [w982 w987] -> w973
              tunnel: w972 -> [w981 w994]
              tunnel: [w981 w986] -> w971
              tunnel: w970 -> [w980 w993]
              tunnel: [w980 w985] -> w969
              tunnel: w968 -> [_ w995]
              tunnel: w967 -> [_ w992]
              tunnel: w966 -> [_ w984]
              frame False {
                n225 = One Button Dialog(message="Stage 1 is not ready") -> ()  [unwired: 1 in, 1 out]
              }
              frame True {
                n226 = flat-sequence {
                  tunnel: w996 -> [w1008]
                  tunnel: w995 -> [w998]
                  tunnel: w994 -> [w1007]
                  tunnel: w993 -> [w1006]
                  tunnel: w992 -> [w1005]
                  tunnel: [w1003] -> w991
                  tunnel: [w1002] -> w990
                  tunnel: [w1001] -> w989
                  tunnel: [w999] -> w988
                  tunnel: w991 -> [w1018]
                  tunnel: w990 -> [w1017]
                  tunnel: w989 -> [w1016]
                  tunnel: w988 -> [w1015]
                  tunnel: [w1014] -> w987
                  tunnel: [w1013] -> w986
                  tunnel: [w1012] -> w985
                  tunnel: w984 -> [w1009]
                  frame #0 {
                    n227 = local read "Axis 2 Velocity (slow)\nmm/s"() -> (w997:dbl)
                    n228 = Concatenate Strings(w998, ".Pos" ("string")) -> (w999:string)
                    n229 = Bundle(cluster=w1005, "Velocity (units/seconds)"=w997) -> (w1004:T2)  [unwired: 3 in]
                    n230 = call <userlib>:"Positioner SGamma Parameters Set.vi"("SGamma Parameters"=w1004, "error in (no error)"=w1006, "XPS error in (no error)"=w1007, "Positioner Name (250 c max)"=w999, "connection ID in"=w1008) -> ("error out"=w1001:errorcluster, "XPS error out"=w1002:errorcluster, "connection ID out"=w1003:T5)  [unwired: 4 in]
                  }
                  frame #1 {
                    n231 = local read "Relative Axis 2"() -> (w1011:dbl)
                    n232 = case shown="True" w1009 {
                      tunnel: w1011 -> [w1019 w1020]
                      tunnel: [w1019 w1021] -> w1010
                      frame False {
                      }
                      frame True {
                        n233 = Negate(x=w1020) -> (-x=w1021:dbl)
                      }
                    }
                    n234 = call <userlib>:"Single Axis Group Move Relative.vi"("Target Displacement (units)"=w1010, "error in (no error)"=w1016, "XPS error in (no error)"=w1017, "SingleAxis Group  Name (250 c max)"=w1015, "connection ID in"=w1018) -> ("error out"=w1012:errorcluster, "XPS error out"=w1013:errorcluster, "connection ID out"=w1014:T5)  [unwired: 4 in]
                  }
                }
              }
            }
          }
        }
      }
      event "Axis 2 move absolute": Value Change {
        n235 = event-data() -> ()  [unwired: 1 in, 6 out]
        n236 = case shown="True" "Axis 2 move absolute" {
          tunnel: w1030 -> [w1033 w1045]
          tunnel: w1027 -> [_ w1044]
          tunnel: w1029 -> [w1032 w1043]
          tunnel: w1028 -> [w1031 w1042]
          tunnel: [w1033 w1040] -> w1024
          tunnel: [w1032 w1038] -> w1023
          tunnel: [w1031 w1036] -> w1022
          tunnel: w1026 -> [_ w1034]
          frame False {
          }
          frame True {
            n237 = call "Stage group check.vi"("error in (no error)"=w1042, "XPS error in (no error)"=w1043, "Group Name (250 c max)"=w1044, "connection ID in"=w1045) -> ("error out"=w1037:errorcluster, "XPS error out"=w1039:errorcluster, "Stages ready?"=w1046:bool, "connection ID out"=w1041:T5, "Group Name (250 c max) 2"=w1035:string)  [unwired: 3 in]
            n238 = case shown="True" w1046 {
              tunnel: w1041 -> [w1049 w1062]
              tunnel: [w1049 w1053] -> w1040
              tunnel: w1039 -> [w1048 w1060]
              tunnel: [w1048 w1052] -> w1038
              tunnel: w1037 -> [w1047 w1059]
              tunnel: [w1047 w1051] -> w1036
              tunnel: w1035 -> [_ w1061]
              tunnel: w1034 -> [_ w1058]
              frame False {
                n239 = One Button Dialog(message="Stage 1 is not ready") -> ()  [unwired: 1 in, 1 out]
              }
              frame True {
                n240 = flat-sequence {
                  tunnel: w1062 -> [w1074]
                  tunnel: w1061 -> [w1063]
                  tunnel: w1060 -> [w1073]
                  tunnel: w1059 -> [w1072]
                  tunnel: w1058 -> [w1071]
                  tunnel: [w1069] -> w1057
                  tunnel: [w1068] -> w1056
                  tunnel: [w1067] -> w1055
                  tunnel: [w1064] -> w1054
                  tunnel: w1057 -> [w1082]
                  tunnel: w1056 -> [w1081]
                  tunnel: w1055 -> [w1080]
                  tunnel: w1054 -> [w1079]
                  tunnel: [w1078] -> w1053
                  tunnel: [w1077] -> w1052
                  tunnel: [w1076] -> w1051
                  frame #0 {
                    n241 = Concatenate Strings(w1063, ".Pos" ("string")) -> (w1064:string)
                    n242 = local read "Axis 2 Velocity (slow)\nmm/s"() -> (w1066:dbl)
                    n243 = Bundle(cluster=w1071, "Velocity (units/seconds)"=w1066) -> (w1070:T2)  [unwired: 3 in]
                    n244 = call <userlib>:"Positioner SGamma Parameters Set.vi"("SGamma Parameters"=w1070, "error in (no error)"=w1072, "XPS error in (no error)"=w1073, "Positioner Name (250 c max)"=w1064, "connection ID in"=w1074) -> ("error out"=w1067:errorcluster, "XPS error out"=w1068:errorcluster, "connection ID out"=w1069:T5)  [unwired: 4 in]
                  }
                  frame #1 {
                    n245 = local read "Absolute Axis 2"() -> (w1075:dbl)
                    n246 = call <userlib>:"Single Axis Group Move Absolute.vi"("Target Position (units)"=w1075, "error in (no error)"=w1080, "XPS error in (no error)"=w1081, "SingleAxis Group  Name (250 c max)"=w1079, "connection ID in"=w1082) -> ("error out"=w1076:errorcluster, "XPS error out"=w1077:errorcluster, "connection ID out"=w1078:T5)  [unwired: 4 in]
                  }
                }
              }
            }
          }
        }
      }
    }
    n247 = call <vilib>:"General Error Handler.vi"("[error source] (\" \")"="Standard" ("[error source] (\" \")"), "error in (no error)"=w172) -> ("error out"=w162:errorcluster)  [unwired: 9 in, 4 out]
    n248 = call <vilib>:"General Error Handler.vi"("[error source] (\" \")"="XPS" ("[error source] (\" \")"), "error in (no error)"=w173) -> ("error out"=w170:errorcluster)  [unwired: 9 in, 4 out]
    n249 = call <vilib>:"Clear Errors.vi"("error in (no error)"=w162, "specific error code to clear (0: all)"=42 ("y")) -> ("error out"=w161:errorcluster)  [unwired: 4 in, 1 out]
    n250 = call <vilib>:"Clear Errors.vi"("error in (no error)"=w170, "specific error code to clear (0: all)"=42 ("y")) -> ("error out"=w164:errorcluster)  [unwired: 4 in, 1 out]
  }
  n251 = property on="Axis 2 Velocity (fast)\nmm/s" class="DigNum (strict)"("Maximum"=w7) -> ()  [unwired: 2 in, 2 out]
  n252 = property on="Axis 2 Velocity (slow)\nmm/s" class="DigNum (strict)"("Maximum"=w7) -> ()  [unwired: 2 in, 2 out]
  n253 = property on="Absolute Axis 2" class="DigNum (strict)"("Data Range"=w4) -> ()  [unwired: 2 in, 2 out]
  n254 = property on="Relative Axis 2" class="DigNum (strict)"("Data Range"=w3) -> ()  [unwired: 2 in, 2 out]
  n255 = property on="Absolute" class="DigNum (strict)"("Data Range"=w2) -> ()  [unwired: 2 in, 2 out]
  n256 = property on="Relative" class="DigNum (strict)"("Data Range"=w1) -> ()  [unwired: 2 in, 2 out]
  n257 = property on="Velocity (slow)" class="DigNum (strict)"("Maximum"=w6) -> ()  [unwired: 2 in, 2 out]
  n258 = property on="Velocity (fast)" class="DigNum (strict)"("Maximum"=w6) -> ()  [unwired: 2 in, 2 out]
